vi "Charger_Is VBAT Complete.vi"(7 "Status Refnum":T1, 8 "error in":errorcluster) -> (0 "error out":errorcluster, 4 "complete":bool)   [LabVIEW 2020]
uses:
  Charger_Status Refnum.ctl
  Drivers/Charger Test Set/Charger_Input Control.ctl
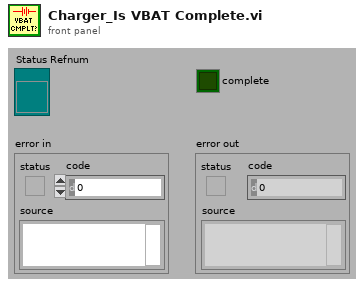
[diagram p1: front panel]
types:
  T1 = typedef "Charger_Status Refnum.ctl" = refnum<vi>
  T2 = typedef "Charger_Input Control.ctl" = cluster{"address":refnum<visa-resource-name>, "position":i32, "setpoint":dbl}
  T3 = cluster{"MICS ID":u32, "VBAT":dbl, "ChargingState":string, "VBAT Slide":dbl, "Status":string, "TemperatureLevel":dbl, "IPG_ReceivedLevel":dbl, "VBAT Target":dbl, "Charger Setpoint":dbl, "Index":i32, "Ready":bool, "Charger Inputs":T2, "MICS Inputs":cluster{"address":refnum<visa-resource-name>, "chan":u16, "ID":u32}}
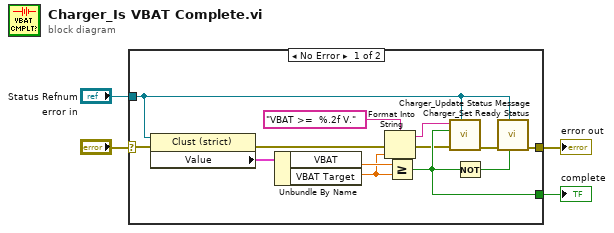
[diagram p0: block diagram]
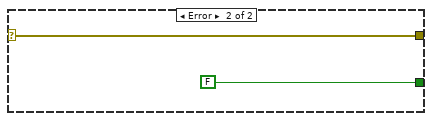
[diagram p2: hidden frame]
diagram:
  n1 = case shown="No Error" "error in" {
    selector: "error in" -> [w10 w19]
    tunnel: "Status Refnum" -> [w6 _]
    tunnel: [w16 w19] -> w3
    tunnel: [w13 FALSE] -> w2
    frame No Error {
      n2 = property on="Status" class="Clust (strict)"(reference=w6, error in=w10) -> (error out=w12:errorcluster, "Value"=w11:T3)  [unwired: 1 out]
      n3 = Unbundle By Name(w11) -> ("VBAT"=w14:dbl, "VBAT Target"=w8:dbl)
      n4 = Format Into String(format string="VBAT >=  %.2f V.", error in=w12, w8) -> (resulting string=w7:string, error out=w9:errorcluster)  [unwired: 1 in]
      n5 = Greater Or Equal?(x=w14, y=w8) -> (x >= y?=w13:bool)
      n6 = call "Charger_Update Status Message.vi"("Status Refnum"=w6, "error in"=w9, "enable (T)"=w13, "status message"=w7) -> ("error out"=w17:errorcluster)  [unwired: 5 in]
      n7 = Not(x=w13) -> (.not. x?=w15:bool)
      n8 = call "Charger_Set Ready Status.vi"("Ready"=w15, "Status Refnum"=w6, "error in"=w17) -> ("error out"=w16:errorcluster)  [unwired: 6 in, 1 out]
    }
    frame Error {
    }
  }
  "error out" <- w3
  "complete" <- w2
